vi "Master Prime Identification (IDN only).vi"(8 "error in (no error)":errorcluster, 10 "VISA resource name":refnum<visa-resource-name>, 11 "Generic Instrument.lvlib:Generic Instrument.lvclass":refnum<class "Generic Instrument.lvclass">) -> (0 "error out":errorcluster, 3 "Generic Instrument out":refnum<class "Generic Instrument.lvclass">)   [LabVIEW 2012, in "Generic Instrument.lvlib" / "Generic Instrument.lvclass"]
uses:
  Generic Instrument.lvclass
  Generic Instrument.lvclass/Generic Instrument.ctl
panel:
  out "VISA resource name 2":refnum<visa-resource-name>
  out "Number of Cards":dbl
  out "ID cluster.Model":string
  out "ID cluster.Manufacturer":string
  out "Instrument ID":string
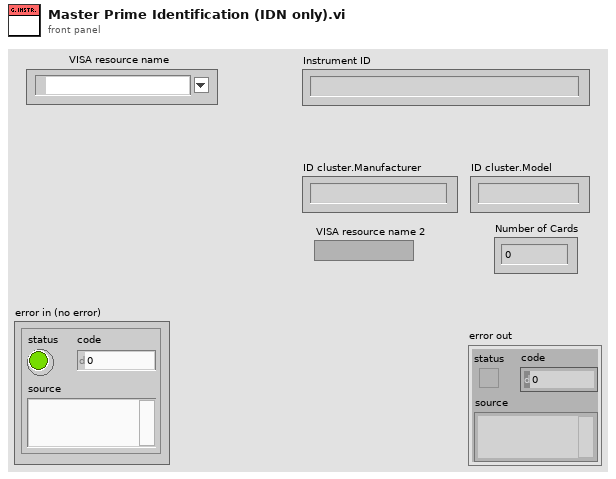
[diagram p1: front panel]
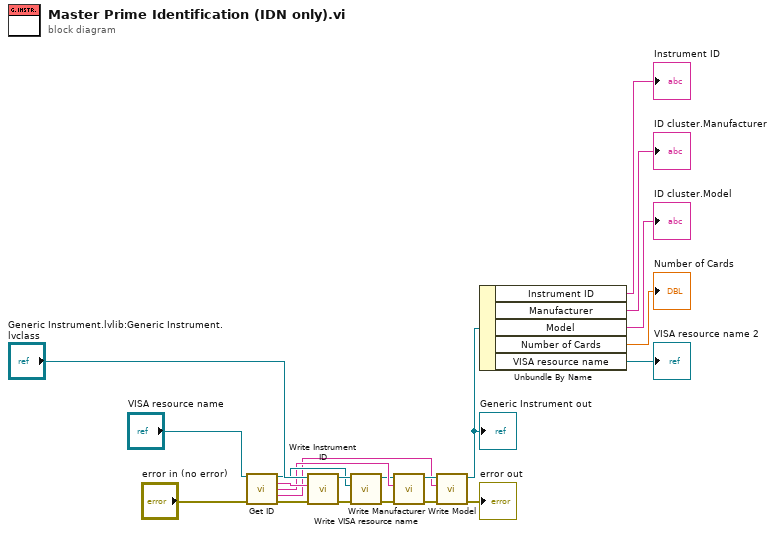
[diagram p0: block diagram]
diagram:
  n1 = call "Get ID.vi"("VISA resource name"="VISA resource name", "error in (no error)"="error in (no error)") -> ("VISA resource name 2"=w17:refnum<visa-resource-name>, "ID"=w19:string, "Manufacturer"=w6:string, "Model"=w5:string, "error out"=w16:errorcluster)  [unwired: 9 in]
  n2 = call-dynamic "Write Instrument ID.vi"("error in (no error)"=w16, "Instrument ID"=w19, "Generic Instrument in"="Generic Instrument.lvlib:Generic Instrument.lvclass") -> ("error out"=w15:errorcluster, "Generic Instrument out"=w18:refnum<class "Generic Instrument.lvclass">)  [unwired: 7 in]
  n3 = call-dynamic "Write VISA resource name.vi"("error in (no error)"=w15, "VISA resource name"=w17, "Generic Instrument in"=w18) -> ("error out"=w2:errorcluster, "Generic Instrument out"=w4:refnum<class "Generic Instrument.lvclass">)  [unwired: 7 in]
  n4 = call "Write Manufacturer.vi"("error in (no error)"=w2, "Manufacturer"=w6, "Generic Instrument in"=w4) -> ("error out"=w7:errorcluster, "Generic Instrument out"=w8:refnum<class "Generic Instrument.lvclass">)  [unwired: 7 in]
  n5 = call "Write Model.vi"("error in (no error)"=w7, "Model"=w5, "Generic Instrument in"=w8) -> ("error out"=→"error out":errorcluster, "Generic Instrument out"=w3:refnum<class "Generic Instrument.lvclass">)  [unwired: 7 in]
  "Generic Instrument out" <- w3
  n6 = Unbundle By Name(w3) -> ("Instrument ID"=→"Instrument ID":string, "Manufacturer"=→"ID cluster.Manufacturer":string, "Model"=→"ID cluster.Model":string, "Number of Cards"=→"Number of Cards":dbl, "VISA resource name"=→"VISA resource name 2":refnum<visa-resource-name>)
